vi "lockin - Set REF phase equals zero.vi"(8 "error in (no error)":errorcluster, 11 "Lockin.DAQ out":refnum<class "Lockin.DAQ.lvclass">) -> (0 "error out":errorcluster, 3 "Lockin.DAQ":refnum<class "Lockin.DAQ.lvclass">)   [LabVIEW 2016, in "Lockin.DAQ.lvclass"]
uses:
  Lockin.DAQ.lvclass
  Lockin.DAQ.lvclass/Lockin.DAQ.ctl
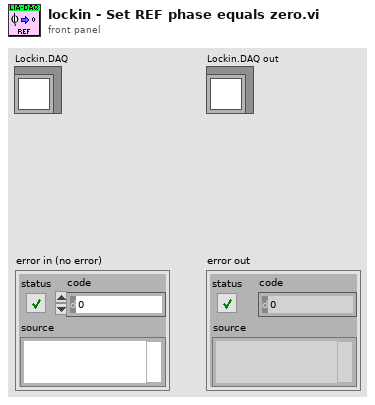
[diagram p1: front panel]
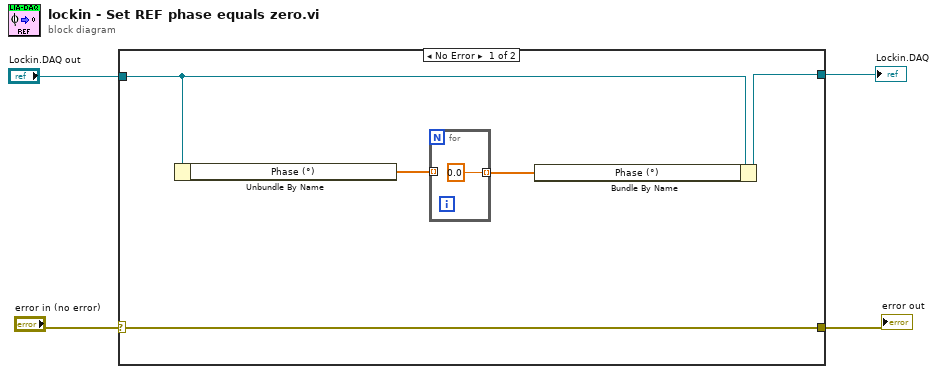
[diagram p0: block diagram]
diagram:
  n1 = case shown="No Error" "error in (no error)" {
    selector: "error in (no error)" -> [w5 w12]
    tunnel: "Lockin.DAQ out" -> [w9 w11]
    tunnel: [w8 w11] -> w3
    tunnel: [w5 w12] -> w1
    frame No Error {
      n2 = Unbundle By Name(w9) -> ("Phase (°)"=w7:dbl[])
      n3 = for {
        tunnel: [0.0] -> w6 mode=indexing
        tunnel: w7 -> [_] mode=indexing
      }
      n4 = Bundle By Name(cluster=w9, "Phase (°)"=w6) -> (w8:refnum<class "Lockin.DAQ.lvclass">)
    }
    frame Error {
    }
  }
  "Lockin.DAQ" <- w3
  "error out" <- w1
